vi "Get App Ini Path.vi"(8 "错误输入":errorcluster) -> (0 "错误输出":errorcluster, 3 "APP.ini":path)   [LabVIEW 2012, in "Application.lvlib"]
uses:
  Application.lvlib
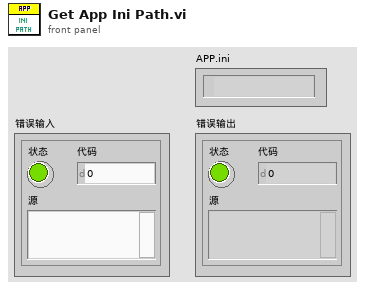
[diagram p1: front panel]
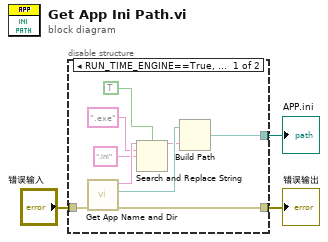
[diagram p0: block diagram]
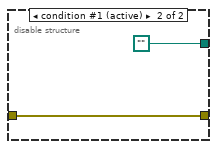
[diagram p2: hidden frame]
diagram:
  n1 = disable-structure shown="RUN_TIME_ENGINE==True, 默认" {
    disable-tunnel: [w6 path ""] -> w3
    disable-tunnel: "错误输入" -> [w5 w13]
    disable-tunnel: [w4 w13] -> w1
    frame condition #0 {
      n2 = call "Get App Name and Dir.vi"("错误输入"=w5) -> ("错误输出"=w4:errorcluster, "AppDir"=w8:path, "AppName"=w12:string)  [unwired: 8 in]
      n3 = Search and Replace String(case sensitive?=TRUE ("忽略大小写？(F)"), input string=w12, search string=".exe" ("搜索字符串"), replace string=".ini" ("替换字符串(\"\")")) -> (result string=w7:string)  [unwired: 4 in, 3 out]
      n4 = Build Path(base path=w8, name or relative path=w7) -> (appended path=w6:path)
    }
    frame condition #1 (active) {
    }
  }
  "APP.ini" <- w3
  "错误输出" <- w1
